vi "GLIMPSE background subtract.vi"(5 "Offset":u8=128, 7 "error in (no error)":errorcluster, 8 "Go ahead":bool, 9 "Output to new directory":path=path "d:/1.glimpse", 10 "Input from existing":path=path "d:/1.glimpse") -> (0 "error out":errorcluster, 3 "Progress":i32(slide) scale=-1.0..182.0)   [LabVIEW 2016]
doc: "Glimpse background subtraction program. Currently supports 8 bit images only."
uses:
  Seq file v 1/Offset table.ctl
  Seq file v 1/Offset.ctl
  Seq file v 1/file number.ctl
  GLIMPSE Globals.vi
  <vilib>/vision/NI_Vision_Development_Module.lvlib
panel:
  out "Bkgd Y Resolution":i32
  out "Bkgd X Resolution":i32
  out "Sequence Y Resolution":i32
  out "Sequence X Resolution":i32
  in  "Abort":bool
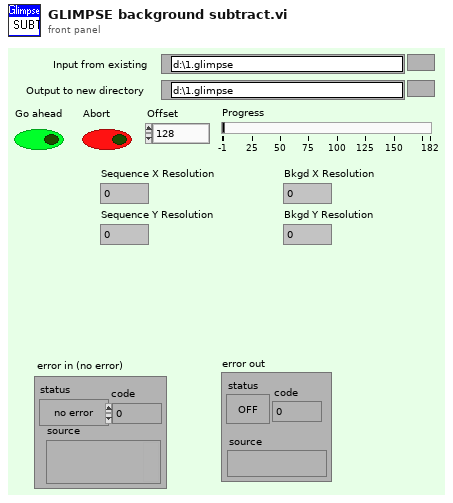
[diagram p1: front panel]
types:
  T1 = enum32{"8 bits", "16 bits", "Float", "Complex", "RGB Chunky", "Compressed"}
  T2 = typedef "Offset table.ctl" = cluster{"offset":T3, "file number":T4}[]
  T3 = typedef "Offset.ctl" = i32
  T4 = typedef "file number.ctl" = u8
  T5 = enum16{"open", "open or create", "create or replace", "create"}
  T6 = typedef "Header2 file data.ctl" = cluster{"Camera":string, "Microscope":string, "Microscope software version":string, "Laser names":string[], "Filter names":string[], "Lasers array":u16[][], "Filter array":u16[], "Flow rate array":dbl[], "Temperature array":dbl[], "Field array":u16[], "Is header2 info present?":bool, "Description Info":string, "Stage xyz array":dbl[][]}
  T7 = typedef "Header file data.ctl" = cluster{"Frames Acquired":u32, "Region width":i32, "Region height":i32, "Element 0 of TTB":u32, "time of 1st frame, \nsec since 1/1/04":dbl, "TTB Array (ms)":u32[], "Offsets Array":T2, "Pixel depth":u32}
  T8 = typedef "Sequence files handle.ctt" = cluster{"Sequence files directory path":path, "Sequence files refnum array":refnum<file>[]}
  T9 = typedef "IMAQ Image.ctl" = refnum<image>
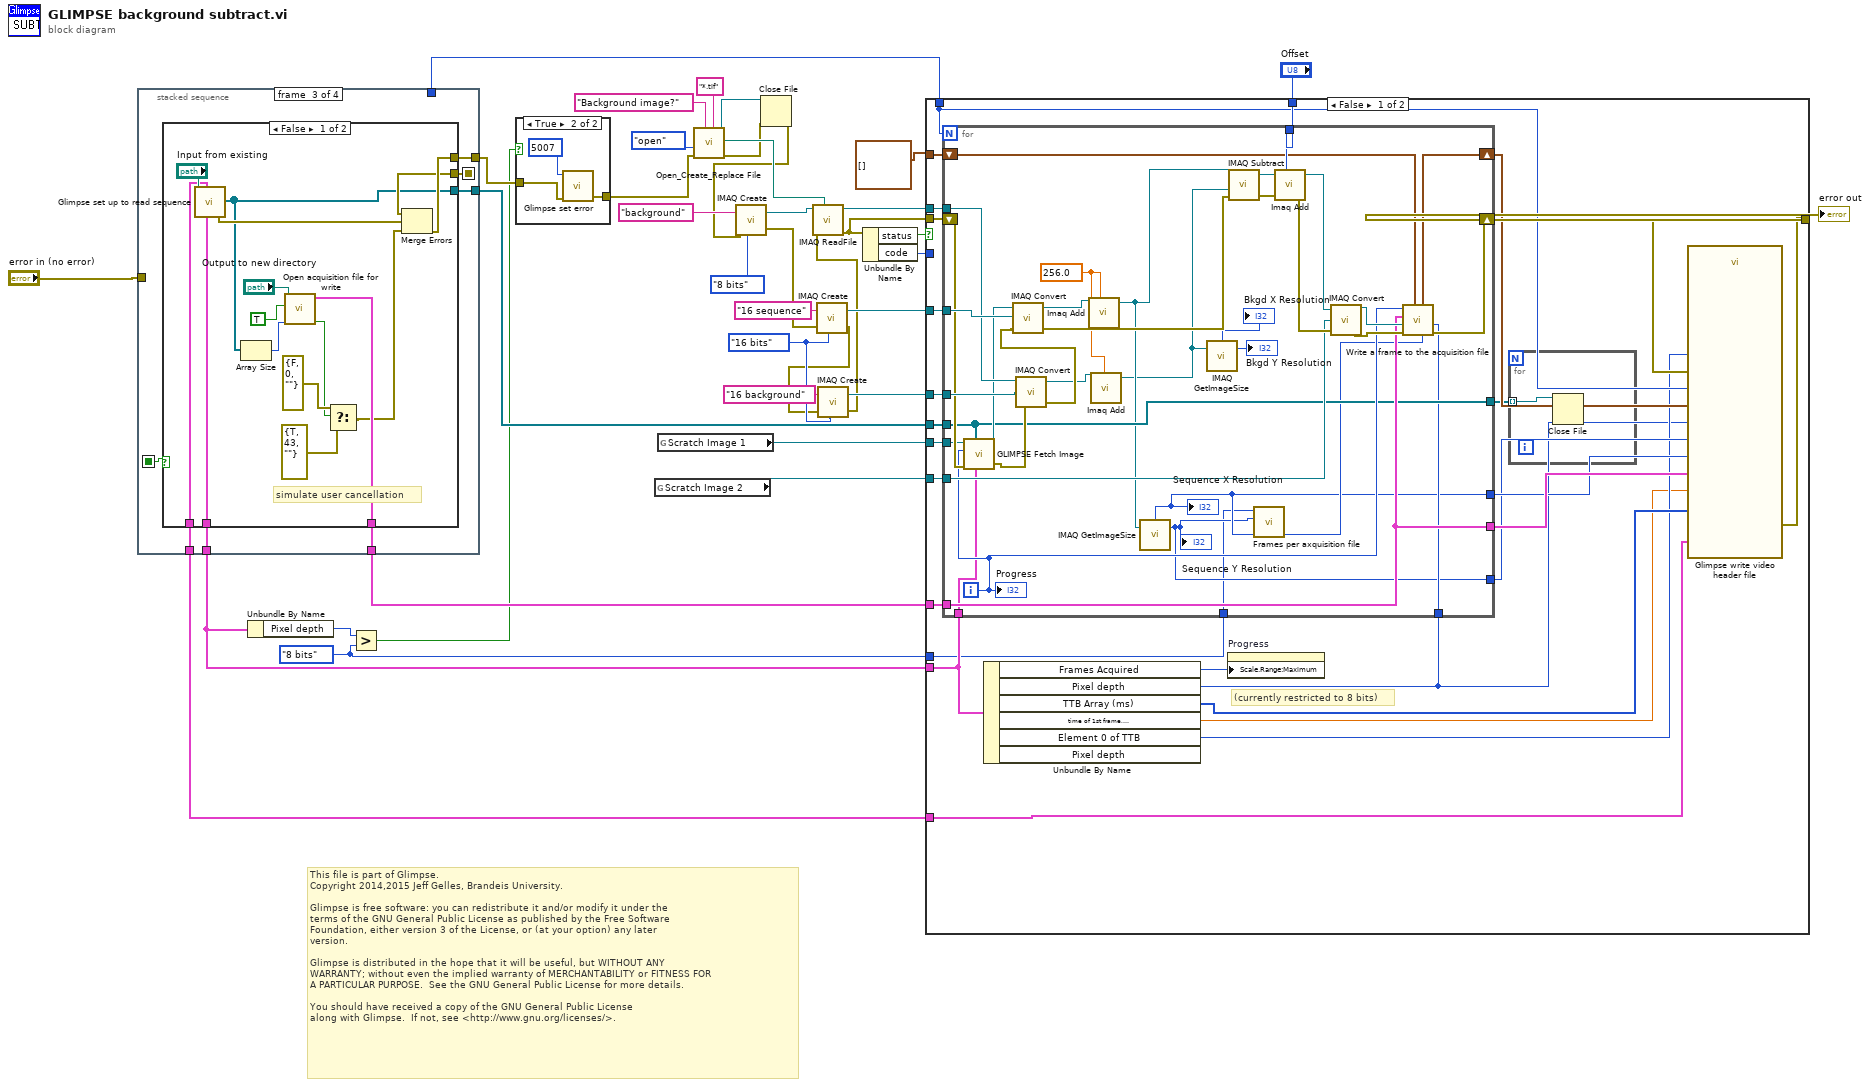
[diagram p0: block diagram]
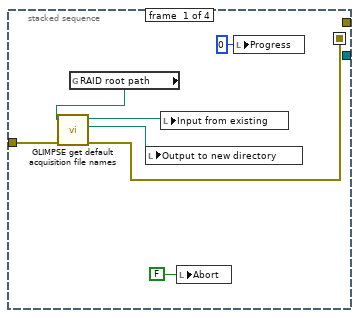
[diagram p3: hidden frame]
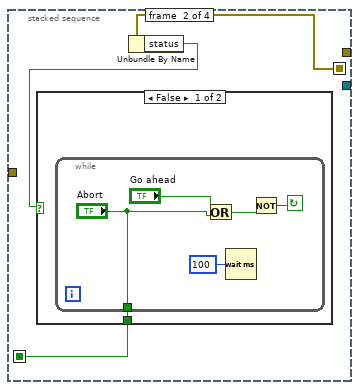
[diagram p4: hidden frame]
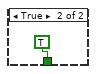
[diagram p5: hidden frame]
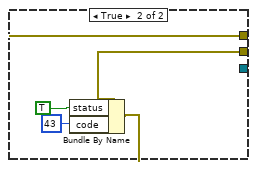
[diagram p6: hidden frame]
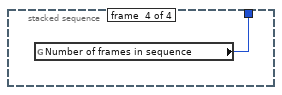
[diagram p7: hidden frame]
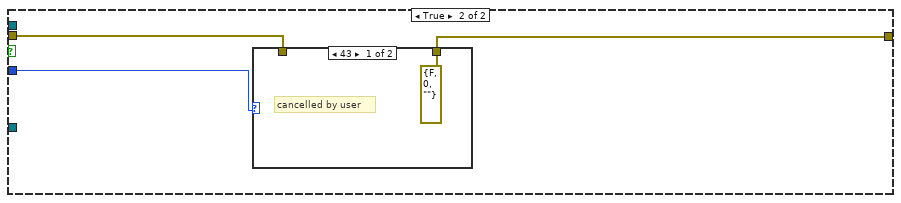
[diagram p8: hidden frame]
diagram:
  w1 = T1."8 bits" ("Image Type")
  w25 = T1."16 bits" ("Image Type")
  # "This file is part of Glimpse. \nCopyright 2014,2015 Jeff Gelles, Brandeis University.    \n\nGlimpse is free software: you can redistribute it and/or modify it under the \nterms of the GNU General Public License as published by the Free Software \nFoundation, either version 3 of the License, or (at your option) any later \nversion.\n\nGlimpse is distributed in the hope that it will be useful, but WITHOUT ANY \nWARRANTY; without even the implied warranty of MERCHANTABILITY or FITNESS FOR \nA PARTICULAR PURPOSE.  See the GNU General Public License for more details.\n\nYou should have received a copy of the GNU General Public License\nalong with Glimpse.  If not, see <http://www.gnu.org/licenses/>."
  n1 = stacked-sequence {
    seq-local: [w40 _ _ _] -> [_ w48 w59 _]
    seq-local: [_ w46 _ _] -> [_ _ w62 _]
    tunnel: "error in (no error)" -> [w43 _ _ _]
    tunnel: [_ _ w61 _] -> w13
    tunnel: [_ _ w60 _] -> w15
    tunnel: [_ _ _ w82] -> w10
    tunnel: [_ _ w58 _] -> w5
    tunnel: [_ _ w57 _] -> w7
    tunnel: [_ _ w56 _] -> w2
    frame #0 {
      n2 = global read "GLIMPSE Globals.vi" "RAID root path"() -> (w44:path)
      n3 = call "GLIMPSE get default acquisition file names.vi"("error in"=w43, "RAID root path"=w44) -> ("error out"=w40:errorcluster, "next directory path"=w42:path, "last directory path"=w41:path)  [unwired: 5 out]
      n4 = local write "Output to new directory"(w42) -> ()
      n5 = local write "Input from existing"(w41) -> ()
      n6 = local write "Abort"(FALSE ("Abort")) -> ()
      n7 = local write "Progress"(i16 0 ("Progress")) -> ()
    }
    frame #1 {
      n8 = Unbundle By Name(w48) -> ("status"=w47:bool)
      n9 = case shown="False" w47 {
        tunnel: [w49 TRUE ("Abort")] -> w46
        frame False {
          n10 = while {
            tunnel: ["Abort"] -> w49
            stop <- w54 continue-if-true
            n11 = Or(x="Go ahead", y="Abort") -> (x .or. y?=w52:bool)
            n12 = Wait (ms)(milliseconds to wait=u32 100) -> ()  [unwired: 1 out]
            n13 = Not(x=w52) -> (.not. x?=w54:bool)
          }
        }
        frame True {
        }
      }
    }
    frame #2 {
      n14 = case shown="False" w62 {
        tunnel: [w74 _] -> w61
        tunnel: [w66 _] -> w60
        tunnel: w59 -> [w72 w81]
        tunnel: [w73 w78] -> w58
        tunnel: [w65 _] -> w57
        tunnel: [w63 _] -> w56
        frame False {
          # "simulate user cancellation"
          n15 = call "Glimpse set up to read sequence.vi"("acquisition directory path"="Input from existing") -> ("Header2 file data out"=w63:T6, "Header file data out"=w65:T7, "Acquisition refnum array"=w66:refnum<file>[], "error out"=w71:errorcluster)  [unwired: 1 in, 2 out]
          n16 = Array Size(array=w66) -> (size(s)=w64:i32)
          n17 = call "Open acquisition file for write.vi"("Number of acquisition files"=w64, "Use new?"=TRUE, "New directory to create"="Output to new directory") -> ("OK?"=w68:bool, "Sequence files handle"=w74:T8)  [unwired: 1 in, 5 out]
          n18 = Select(t=errorcluster {"status"=FALSE, "code"=0, "source"=""} ("error in 3 (no error)"), s=w68, f=errorcluster {"status"=TRUE, "code"=43, "source"=""} ("error in 3 (no error)")) -> (s? t:f=w67:errorcluster)
          n19 = Merge Errors(w72, w71, w67) -> (w73:errorcluster)
        }
        frame True {
          n20 = Bundle By Name(cluster=w81, "status"=TRUE, "code"=43) -> (w78:errorcluster)
        }
      }
    }
    frame #3 {
      n21 = global read "GLIMPSE Globals.vi" "Number of frames in sequence"() -> (w82:u32)
    }
  }
  n22 = Unbundle By Name(w7) -> ("Pixel depth"=w6:u32)
  n23 = Greater?(x=w6, y=w1) -> (0:w3:bool)
  n24 = case shown="True" w3 {
    tunnel: w5 -> [w83 w85]
    tunnel: [w83 w84] -> w4
    frame False {
    }
    frame True {
      n25 = call "Glimpse set error.vi"("code"=5007, "error in"=w85) -> ("error out"=w84:errorcluster)  [unwired: 1 in, 5 out]
    }
  }
  n26 = global read "GLIMPSE Globals.vi" "Scratch Image 2"() -> (w14:T9)
  n27 = global read "GLIMPSE Globals.vi" "Scratch Image 1"() -> (w16:T9)
  n28 = call <vilib>:"Open_Create_Replace File.vi"("pattern"="*.tif", "prompt"="Background image?", "error in (no error)"=w4, "function (open:0)"=T5."open") -> ("error out"=w27:errorcluster, "new file path"=w32:path, "refnum"=w28:refnum<file>)  [unwired: 3 in, 2 out]
  n29 = Close File(refnum=w28, error in=w27) -> (error out=w26:errorcluster)  [unwired: 1 out]
  n30 = call "IMAQ Create"("Image Name"="background", "Image Type"=T1."8 bits", "error in (no error)"=w26) -> ("New Image"=w38:T9, "error out"=w19:errorcluster)  [unwired: 1 in, 1 out]
  n31 = call "IMAQ Create"("Image Name"="16 sequence", "Image Type"=w25, "error in (no error)"=w19) -> ("New Image"=w22:T9, "error out"=w20:errorcluster)  [unwired: 1 in, 1 out]
  n32 = call "IMAQ Create"("Image Name"="16 background", "Image Type"=w25, "error in (no error)"=w20) -> ("New Image"=w21:T9, "error out"=w18:errorcluster)  [unwired: 1 in, 1 out]
  n33 = call "IMAQ ReadFile"("File Path"=w32, "error in (no error)"=w18, "Image"=w38) -> ("error out"=w11:errorcluster, "Image Out"=w35:T9)  [unwired: 2 in, 5 out]
  n34 = Unbundle By Name(w11) -> ("status"=w29:bool, "code"=w9:i32)
  n35 = case shown="False" w29 {
    tunnel: w35 -> [w112 _]
    tunnel: w11 -> [w111 w150]
    tunnel: [w98 w151] -> w34
    tunnel: "Offset" -> [w110 _]
    tunnel: w22 -> [w109 _]
    tunnel: w21 -> [w108 _]
    tunnel: w16 -> [w107 _]
    tunnel: w15 -> [w106 _]
    tunnel: w14 -> [w105 _]
    tunnel: w13 -> [w104 _]
    tunnel: T2 [] ("Offset table out") -> [w103 _]
    tunnel: w10 -> [w97 _]
    tunnel: w9 -> [_ w152]
    tunnel: w7 -> [w96 _]
    tunnel: w2 -> [w88 _]
    tunnel: w1 -> [w87 _]
    frame False {
      # "(currently restricted to 8 bits)"
      n36 = Unbundle By Name(w96) -> ("Frames Acquired"=w95:u32, "Pixel depth"=w90:u32, "TTB Array (ms)"=w94:u32[], "time of 1st frame, \nsec since 1/1/04"=w89:dbl, "Element 0 of TTB"=w91:u32)  [unwired: 1 out]
      n37 = for {
        N: w97 -> [_]
        tunnel: w112 -> [w144]
        shift-right: [w130] -> w101
        shift-left: w111 -> [w134]
        tunnel: w110 -> [w147]
        tunnel: w109 -> [w146]
        tunnel: w108 -> [w145]
        tunnel: w107 -> [w133]
        tunnel: w106 -> [w124]
        tunnel: w105 -> [w132]
        tunnel: w104 -> [w125]
        shift-right: [w127] -> w102
        shift-left: w103 -> [w126]
        tunnel: [w125] -> w100
        tunnel: [w124] -> w99
        tunnel: w96 -> [w119]
        tunnel: w90 -> [w117]
        tunnel: [w116] -> w93
        tunnel: [w115] -> w92
        tunnel: w87 -> [w114]
        i -> [w128]
        w139 = sgl 256.0 ("Constant")
        n38 = call "GLIMPSE Fetch Image.vi"("Header file data"=w119, "Acqisition files refnums"=w124, "error in"=w134, "Logical Frame Number\n(starting with zero)"=w128, "Image In"=w133) -> ("error out"=w135:errorcluster, "Image Out"=w136:T9)  [unwired: 2 in, 3 out]
        n39 = call "IMAQ Convert"("error in (no error)"=w135, "Image Dst"=w145, "Image Src"=w144) -> ("error out"=w143:errorcluster, "Image Dst Out"=w141:T9)  [unwired: 1 out]
        n40 = call "IMAQ Convert"("error in (no error)"=w143, "Image Dst"=w146, "Image Src"=w136) -> ("error out"=w142:errorcluster, "Image Dst Out"=w140:T9)  [unwired: 1 out]
        n41 = call "Imaq Add"("Image Src A"=w140, "Constant"=w139) -> ("Image Dst Out"=w123:T9)  [unwired: 3 in, 3 out]
        n42 = call "Imaq Add"("Image Src A"=w141, "Constant"=w139) -> ("Image Dst Out"=w122:T9)  [unwired: 3 in, 3 out]
        n43 = call "IMAQ GetImageSize"("Image"=w123) -> ("Y Resolution"=w115:i32, "X Resolution"=w116:i32)  [unwired: 1 in, 3 out]
        "Sequence X Resolution" <- w116
        "Sequence Y Resolution" <- w115
        n44 = call "IMAQ GetImageSize"("Image"=w122) -> ("Y Resolution"=→"Bkgd Y Resolution":i32, "X Resolution"=→"Bkgd X Resolution":i32)  [unwired: 1 in, 3 out]
        n45 = call "IMAQ Subtract"("Image Src A"=w123, "Image Src B"=w122, "error in (no error)"=w142) -> ("Image Dst Out"=w148:T9, "error out"=w149:errorcluster)  [unwired: 2 in, 2 out]
        n46 = call "Frames per axquisition file.vi"("Output frame width"=w116, "Output frame height"=w115, "Pixel depth"=w114) -> ("Frames per acquisition file"=w118:i32)  [unwired: 3 in, 1 out]
        n47 = call "Imaq Add"("Image Src A"=w148, "Constant"=w147, "error in (no error)"=w149) -> ("Image Dst Out"=w137:T9, "error out"=w138:errorcluster)  [unwired: 2 in, 2 out]
        n48 = call "IMAQ Convert"("error in (no error)"=w138, "Image Dst"=w132, "Image Src"=w137) -> ("error out"=w131:errorcluster, "Image Dst Out"=w129:T9)  [unwired: 1 out]
        n49 = call "Write a frame to the acquisition file.vi"("Pixel depth"=w117, "Frames per acquisition file"=w118, "Offset table in"=w126, "error in"=w131, "Image In"=w129, "Sequence files handle"=w125, "Last frame number written in"=w128) -> ("error out"=w130:errorcluster, "Offset table out"=w127:T2)  [unwired: 3 out]
        "Progress" <- w128
      }
      n50 = property on="Progress" class="Slide (strict)"("Scale.Range:Maximum"=w95) -> ()  [unwired: 2 in, 2 out]
      n51 = for {
        tunnel: w99 -> [w113] mode=indexing
        n52 = Close File(refnum=w113) -> ()  [unwired: 1 in, 2 out]
      }
      n53 = call "Glimpse write video header file.vi"("Number of frames"=w97, "Sequence files handle"=w100, "Pixel depth\n(0=8 bit; 1= 16 bit)"=w90, "error in"=w101, "TTB Array"=w94, "Offsets Array"=w102, "Header2 file data"=w88, "Region width"=w93, "Region height"=w92, "Element 0 of TTB"=w91, "time of 1st frame, \nsec since 1/1/04"=w89) -> ("error out"=w98:errorcluster)  [unwired: 8 in]
    }
    frame True {
      n54 = case shown="43" w152 {
        tunnel: [errorcluster {"status"=FALSE, "code"=0, "source"=""} ("error out") w154] -> w151
        tunnel: w150 -> [_ w154]
        frame 43 {
          # "cancelled by user"
        }
        frame 1, Default {
        }
      }
    }
  }
  "error out" <- w34
